vi "Exchange Connection Names.vi"(8 "error in (no error)":errorcluster, 10 "This Connection Name in":string, 11 "connection ID":refnum<k5>) -> (0 "error out":errorcluster, 1 "Message Priority":T1=enum."Normal", 2 "Remote Connection Name out":string, 3 "connection out":refnum<k5>)   [LabVIEW 2017, in "DS TCP Server.lvlib" / "DS TCP Listener.lvclass"]
uses:
  DS TCP Listener.lvclass
  <vilib>/addons/_Workers/Library/Classes/Message/Priority.ctl
  <vilib>/addons/_Workers/Library/Classes/Message/Message.lvclass
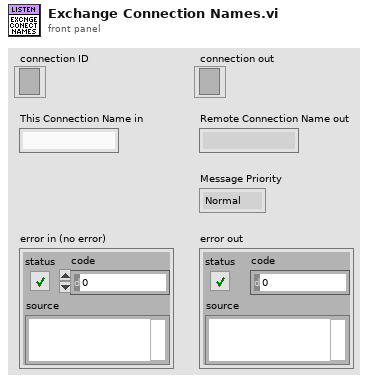
[diagram p1: front panel]
types:
  T1 = typedef "Workers.lvlib/Message.lvclass/Priority.ctl" = enum16{"Low", "Normal", "High"}
  T2 = enum16{"Standard", "Buffered", "CRLF", "Immediate"}
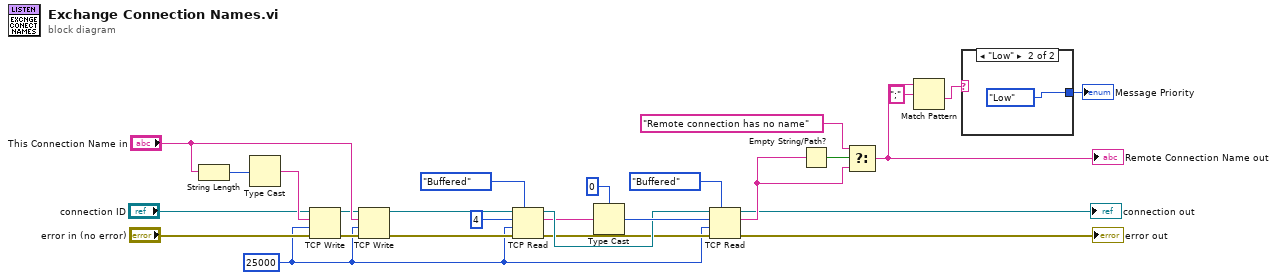
[diagram p0: block diagram]
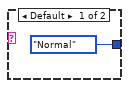
[diagram p2: hidden frame]
diagram:
  w1 = 25000 ("timeout ms (25000)")
  n1 = String Length(string="This Connection Name in") -> (length=w26:i32)
  n2 = Type Cast(x=w26) -> (*(type *) &x=w25:string)  [unwired: 1 in]
  n3 = TCP Write(connection ID="connection ID", data in=w25, error in (no error)="error in (no error)", 9:w1) -> (connection ID out=w23:refnum<k5>, error out=w24:errorcluster)  [unwired: 1 out]
  n4 = TCP Write(connection ID=w23, data in="This Connection Name in", error in (no error)=w24, 9:w1) -> (connection ID out=w10:refnum<k5>, error out=w3:errorcluster)  [unwired: 1 out]
  n5 = TCP Read(connection ID=w10, bytes to read=4, error in (no error)=w3, 7:T2."Buffered" ("mode (standard)"), 9:w1) -> (connection ID out=w15:refnum<k5>, data out=w14:string, error out=w12:errorcluster)
  n6 = Type Cast(type=0 ("bytes to read"), x=w14) -> (*(type *) &x=w18:i32)
  n7 = TCP Read(connection ID=w15, bytes to read=w18, error in (no error)=w12, 7:T2."Buffered" ("mode (standard)"), 9:w1) -> (connection ID out=→"connection out":refnum<k5>, data out=w21:string, error out=→"error out":errorcluster)
  n8 = Empty String/Path?(string/path=w21) -> (empty?=w19:bool)
  n9 = Select(t="Remote connection has no name", s=w19, f=w21) -> (s? t:f=w7:string)
  "Remote Connection Name out" <- w7
  n10 = Match Pattern(string=w7, regular expression=";") -> (after substring=w5:string)  [unwired: 1 in, 3 out]
  n11 = case shown="\"Low\"" w5 {
    tunnel: [Priority."Normal" ("Message Priority") Priority."Low" ("Message Priority")] -> w4
    frame Default {
    }
    frame "Low" {
    }
  }
  "Message Priority" <- w4
